vi "PhasedArrayRadar.vi"() -> ()   [LabVIEW 2015]
doc: "This example demonstrates how to use the Short-time Fourier Transform (STFT Spectrograms) VI to analyze the Time-Frequency spectrogram."
uses:
  <vilib>/Math Plots/3D Math Plots/3D Surface/3D Surface XCtrl/3D Surface.xctl
  <vilib>/sound2/lvsound2.llb/Sampling Mode.ctl
  <vilib>/Analysis/baseanly.llb/Mean (DBL).vi
  <vilib>/Analysis/2dsp.llb/Real FFT.vi
  <vilib>/Utility/file.llb/Read Delimited Spreadsheet (I64).vi
  <vilib>/Analysis/Matrix/Numeric/Conversions/Array To Matrix - RA.vi
  <vilib>/Analysis/Matrix/Numeric/Multiply/Multiply - RM,RM.vi
  <vilib>/Analysis/Matrix/Numeric/Conversions/Matrix To Array - RM.vi
  <vilib>/sound2/lvsound2.llb/Sound Input Read (DBL).vi
  <vilib>/Math Plots/3D Math Plots/3D Surface/3D Surface Datatype/Public/Plot Helper (Matrix).vi
  <vilib>/Analysis/NI_AALPro.lvlib
  <vilib>/Analysis/NI_AALBase.lvlib
  <vilib>/Math Plots/3D Math Plots/3D Surface/3D Surface Datatype/3D Surface Datatype.lvclass
  <vilib>/Analysis/Matrix/NI_Matrix.lvlib
panel:
  in  "Chirp repetition frequency":dbl=124.0
  in  "Save processed data":bool
  in  "Save raw data":bool
  in  "Data saving path":path=path "C:/Users/zpeng/OneDrive - Texas Tech University/Desktop/BeamSteering/data"
  out "3D Surface":refnum<class "3D Plot Datatype.lvclass">[](xcontrol)
  in  "Beam steering calibration data path":path=path "C:/Users/zpeng/OneDrive - Texas Tech University/Desktop/BeamSteering/voltages"
  in  "Angle step":dbl=2.5
  in  "Angle start":dbl=-60.0
  in  "Angle stop":dbl=60.0
  in  "Duty ratio":dbl=0.4
  in  "begin offsets":i32=548
  in  "end offsets":i32=562
  in  "Range":dbl(slide)=5.101767831965583 min=1.0 max=77.41935483870968 scale=0.0..77.41935483870968
  out "Range resolution":dbl
  in  "Bandwidth (MHz)":dbl=600.0
  in  "Range intensify:Minimum":dbl=-40.0
  out "Chirp frequency":dbl
  in  "FFT length":i32=4096
  out "Samples per chirp":i32
  in  "threshold":dbl=0.6 format="%0.2f"
  in  "Sample rate (S/s)":dbl=192000.0
  in  "Samples per read":i32=40000 min=1024 max=100000
  in  "Device ID":u32
  # "Phased Array"
  # "Version: 3\nZhengyu Peng\nC. Li Lab\nTexas Tech University\nJan. 2016"
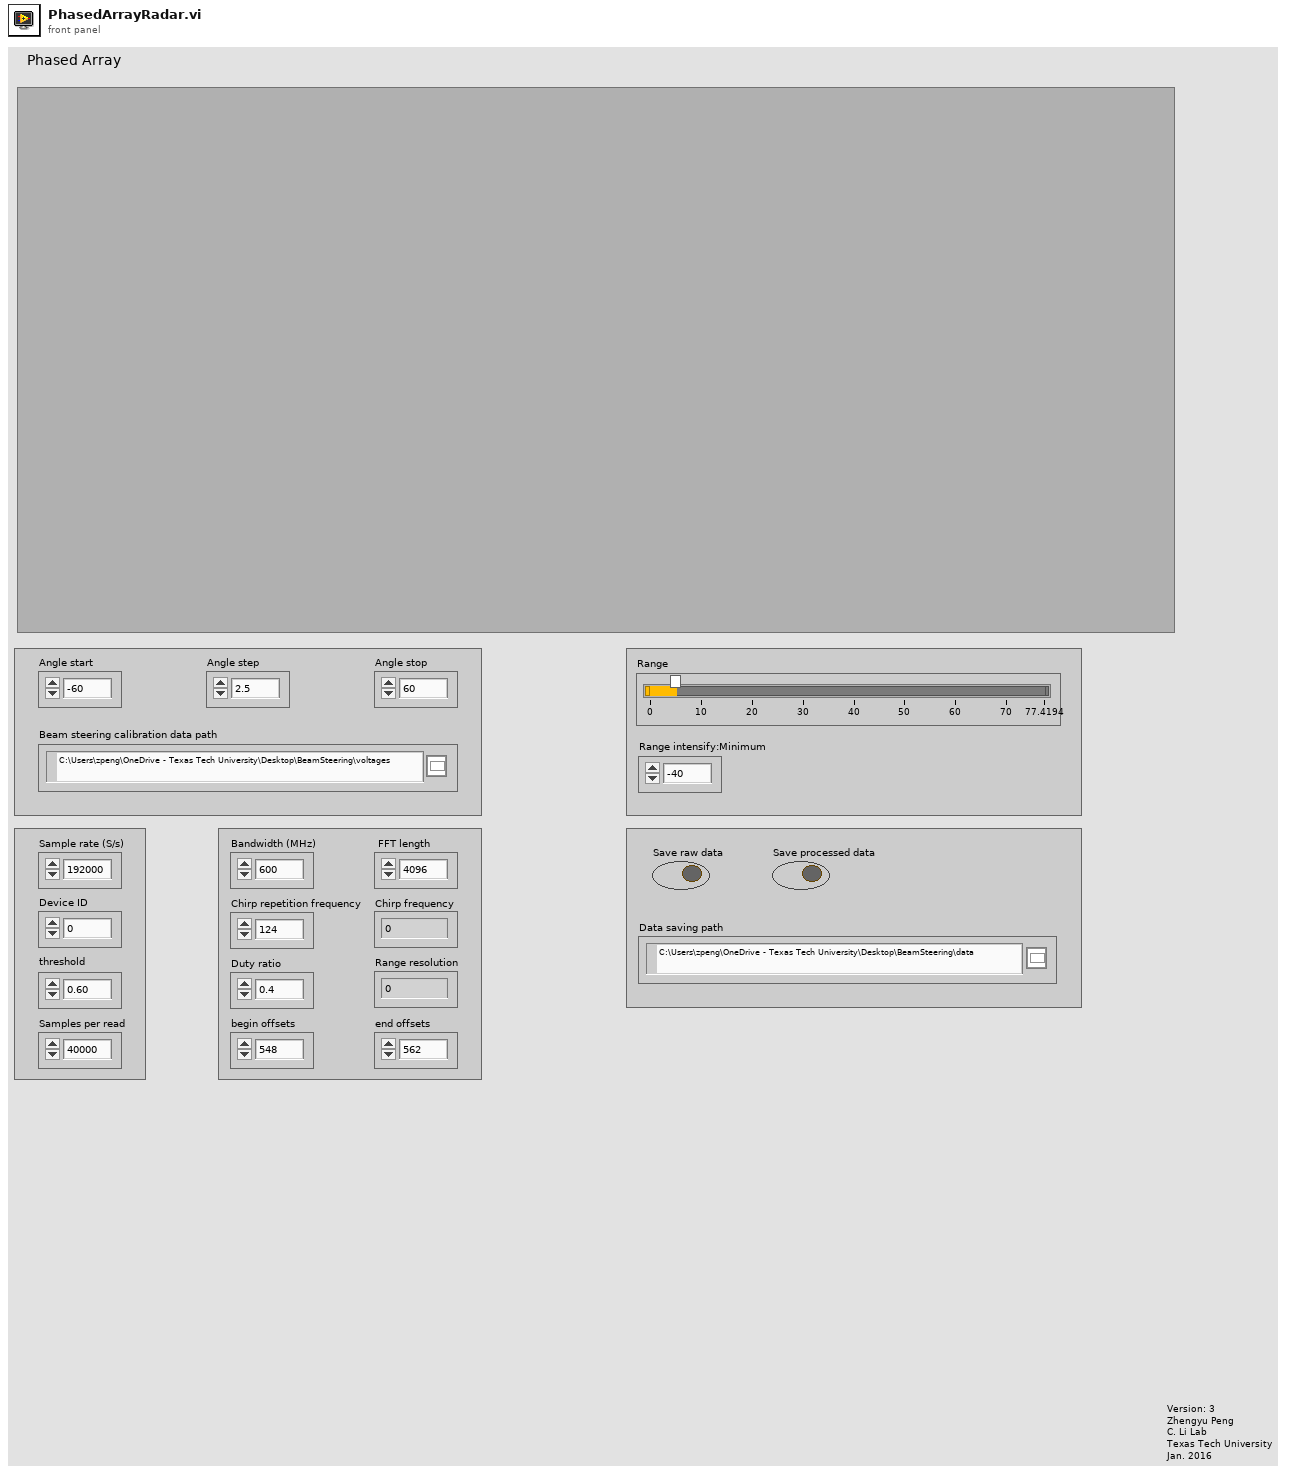
[diagram p1: front panel]
types:
  T1 = cluster{"Sample rate (S/s)":dbl, "number of channels":i32, "bits per sample":i32}
  T2 = typedef "NI_Matrix.lvlib/RealMatrix.ctl" = dbl[][]
  T3 = typedef "Sampling Mode.ctl" = i32
  T4 = typedef "Sound Input Task ID.ctl" = u32
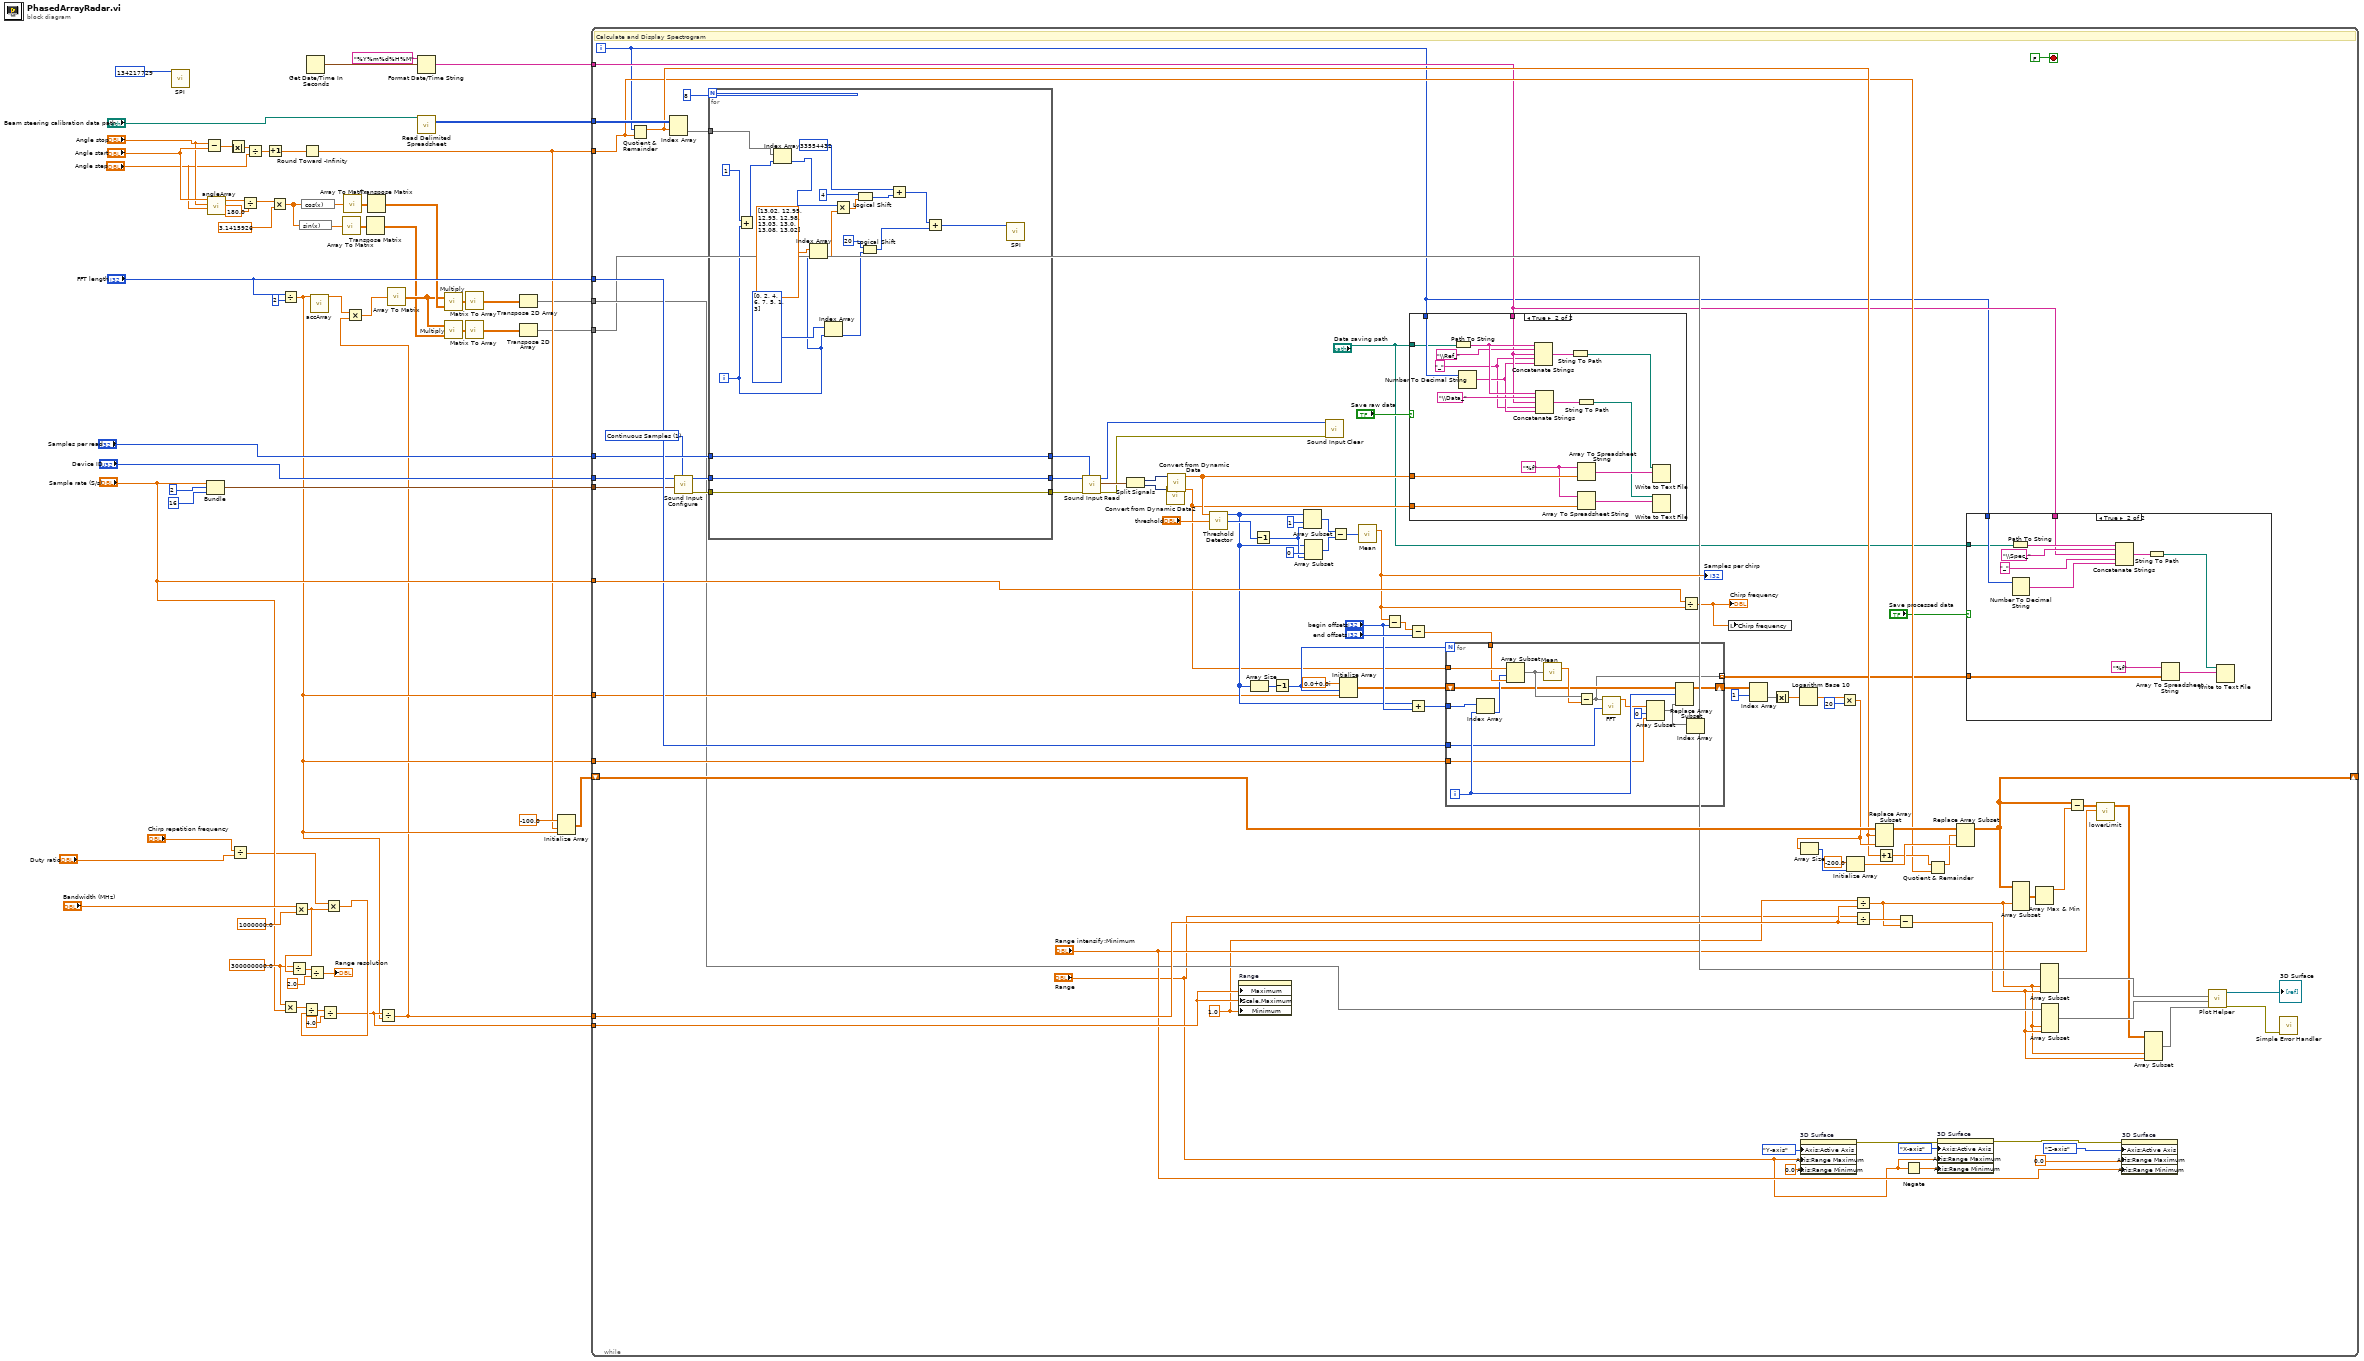
[diagram p0: block diagram]
diagram:
  w54 = 300000000.0 ("x")
  n1 = call "SPI.vi"("data"=u32 134217729) -> ()  [unwired: 11 in]
  n2 = Subtract(x="Angle stop", y="Angle start") -> (x-y=w41:dbl)
  n3 = Bundle("Sample rate (S/s)"="Sample rate (S/s)", "number of channels"=2, "bits per sample"=16) -> (w33:T1)  [unwired: 1 in]
  n4 = call "angleArray.vi"("Angle step"="Angle step", "Angle stop"="Angle stop", "Angle start"="Angle start") -> ("Array"=w26:dbl[])  [unwired: 8 in]
  n5 = Absolute Value(x=w41) -> (abs(x)=w40:dbl)
  n6 = Divide(x="Chirp repetition frequency", y="Duty ratio") -> (x/y=w45:dbl)
  n7 = Divide(x=w26, y=180.0) -> (x/y=w24:dbl[])
  n8 = Divide(x=w40, y="Angle step") -> (x/y=w39:dbl)
  n9 = Increment(x=w39) -> (x+1=w38:dbl)
  n10 = Multiply(x=w24, y=3.1415926) -> (x*y=w22:dbl[])
  n11 = Divide(x="FFT length", y=2) -> (x/y=w27:dbl)
  n12 = Multiply(x=w54, y="Sample rate (S/s)") -> (x*y=w53:dbl)
  n13 = Multiply(x="Bandwidth (MHz)", y=1000000.0) -> (x*y=w58:dbl)
  n14 = Divide(x=w54, y=w58) -> (x/y=w57:dbl)
  n15 = expression code="sin(x)"(w22) -> (w20:dbl[])
  n16 = expression code="cos(x)"(w22) -> (w21:dbl[])
  n17 = Round Toward -Infinity(1:w38) -> (0:w31:dbl)
  n18 = Get Date/Time In Seconds() -> (seconds since 1Jan1904=w4:timestamp)
  n19 = Divide(x=w57, y=2.0) -> (x/y=→"Range resolution":dbl)
  n20 = call "accArray.vi"("data length"=w27) -> ("Array"=w7:dbl[])  [unwired: 10 in]
  n21 = Multiply(x=w45, y=w58) -> (x*y=w52:dbl)
  n22 = Divide(x=w53, y=w52) -> (x/y=w51:dbl)
  n23 = Divide(x=w51, y=4.0) -> (x/y=w46:dbl)
  n24 = call-poly <vilib>:"Array To Matrix.vi"("Real 1D Array"=w20) -> ("Real Matrix (Column Vector)"=w18:T2)
  n25 = call-poly <vilib>:"Array To Matrix.vi"("Real 1D Array"=w21) -> ("Real Matrix (Column Vector)"=w19:T2)
  n26 = Transpose Matrix(1:w18) -> (0:w15:T2)
  n27 = Transpose Matrix(1:w19) -> (0:w17:T2)
  n28 = Divide(x=w46, y=w27) -> (x/y=w8:dbl)
  n29 = Multiply(x=w7, y=w8) -> (x*y=w6:dbl[])
  n30 = call-poly <vilib>:"Array To Matrix.vi"("Real 1D Array"=w6) -> ("Real Matrix (Column Vector)"=w16:T2)
  n31 = Format Date/Time String(time format string (%c)="%Y%m%d%H%M", seconds (now)=w4) -> (date/time string=w2:string)  [unwired: 1 in]
  n32 = call-poly <vilib>:"Read Delimited Spreadsheet.vi"("file path (dialog if empty)"="Beam steering calibration data path") -> ("all rows"=w35:i64[][])  [unwired: 9 in, 5 out]
  n33 = call-poly <vilib>:"Multiply.vi"("Real Matrix B"=w17, "Real Matrix A"=w16) -> ("A * B"=w14:T2)
  n34 = call-poly <vilib>:"Multiply.vi"("Real Matrix B"=w15, "Real Matrix A"=w16) -> ("A * B"=w13:T2)
  n35 = call-poly <vilib>:"Matrix To Array.vi"("Real Matrix"=w14) -> ("Real 2D Array"=w12:dbl[][])
  n36 = call-poly <vilib>:"Matrix To Array.vi"("Real Matrix"=w13) -> ("Real 2D Array"=w10:dbl[][])
  n37 = Transpose 2D Array(2D array=w12) -> (transposed array=w11:dbl[][])
  n38 = Transpose 2D Array(2D array=w10) -> (transposed array=w9:dbl[][])
  n39 = Initialize Array(-100.0 ("element"), w31, w27) -> (w32:dbl[][])
  n40 = while {
    tunnel: "Device ID" -> [w115]
    tunnel: "Samples per read" -> [w120]
    tunnel: "Sample rate (S/s)" -> [w142]
    tunnel: "FFT length" -> [w141]
    tunnel: w8 -> [w106]
    tunnel: w27 -> [w140]
    tunnel: w46 -> [w139]
    tunnel: w27 -> [w127]
    tunnel: w31 -> [w77]
    tunnel: w35 -> [w122]
    shift-right: [w79] -> _
    shift-left: w32 -> [w116]
    tunnel: w33 -> [w112]
    tunnel: w11 -> [w104]
    tunnel: w9 -> [w103]
    tunnel: w2 -> [w65]
    i -> [w64]
    stop <- FALSE stop-if-true
    w72 = T3 1 items=["Finite Samples", "Continuous Samples"] ("sample mode")
    w86 = 1.0 ("Data Entry Limits:Minimum")
    # "Calculate and Display Spectrogram"
    n41 = Quotient & Remainder(x=w64, y=w77) -> (x-y*floor(x/y)=w81:dbl)  [unwired: 1 out]
    n42 = Index Array(array=w122, index (row)=w81) -> (element=w123:i64[])  [unwired: 1 in]
    n43 = call <vilib>:"Sound Input Configure.vi"("sample mode"=w72, "sound format"=w112, "device ID"=w115) -> ("error out"=w113:errorcluster, "task ID"=w114:T4)  [unwired: 7 in]
    n44 = for {
      N: 8 -> [_]
      tunnel: w123 -> [w194]
      tunnel: [w187] -> w121
      tunnel: w114 -> [w187]
      tunnel: [w186] -> w119
      tunnel: w120 -> [w186]
      tunnel: [w185] -> w118
      tunnel: w113 -> [w185]
      i -> [w188]
      n45 = Add(x=1 ("length"), y=w188) -> (x+y=w193:i32)
      n46 = Index Array(array=w194, index=w193) -> (element=w192:i64)
      n47 = Index Array(array=dbl[] [13.02, 12.95, 12.93, 12.98, 13.03, 13.0, 13.08, 13.02] ("y"), index=w188) -> (element=w189:dbl)
      n48 = Index Array(array=i32[] [0, 2, 4, 6, 7, 5, 1, 3], index=w188) -> (element=w191:i32)
      n49 = Multiply(x=w192, y=w189) -> (x*y=w198:dbl)
      n50 = Logical Shift(y=u32 4 ("x"), x=w198) -> (x << y=w203:u32)
      n51 = Logical Shift(y=u32 20 ("x"), x=w191) -> (x << y=w201:i32)
      n52 = Add(x=u32 33554432 ("y"), y=w203) -> (x+y=w202:u32)
      n53 = Add(x=w202, y=w201) -> (x+y=w200:u32)
      n54 = call "SPI.vi"("data"=w200) -> ()  [unwired: 11 in]
    }
    n55 = call-poly <vilib>:"Sound Input Read.vi"("number of samples/ch"=w119, "error in (no error)"=w118, "task ID"=w121) -> ("error out"=w108:errorcluster, "data"=w153:waveform(dbl)[], "task ID out"=w111:T4)  [unwired: 6 in]
    n56 = Split Signals(w153) -> (w155:dynamicdata, w154:dynamicdata)  [unwired: 2 out]
    n57 = call "Convert from Dynamic Data2"("Dynamic Data Type"=w154) -> ("Array"=w69:dbl[])  [unwired: 3 out]
    n58 = call "Convert from Dynamic Data"("Dynamic Data Type"=w155) -> ("Array"=w70:dbl[])  [unwired: 3 out]
    n59 = call <vilib>:"Threshold Detector.vi"("threshold"="threshold", "X"=w70) -> ("count"=w148:i32, "Indices"=w131:i32[])  [unwired: 1 in, 1 out]
    n60 = property on="Range" class="Slide (strict)"("Maximum"=w139, "Scale.Maximum"=w139, "Minimum"=w86) -> ()  [unwired: 2 in, 2 out]
    n61 = Array Size(array=w131) -> (size(s)=w130:i32)
    n62 = Decrement(x=w148) -> (x-1=w147:i32)
    n63 = Decrement(x=w130) -> (x-1=w128:i32)
    n64 = Array Subset(array=w131, index=1, length=w147) -> (w150:i32[])
    n65 = Array Subset(array=w131, index=0, length=w147) -> (w149:i32[])
    n66 = call <vilib>:"Sound Input Clear.vi"("error in (no error)"=w108, "task ID"=w111) -> ()  [unwired: 9 in, 1 out]
    n67 = Subtract(x=w150, y=w149) -> (x-y=w146:i32[])
    n68 = Initialize Array(cdb 0.0+0.0i ("element"), w128, w127) -> (w126:cdb[][])
    n69 = call-poly <vilib>:"Mean.vi"("X"=w146) -> ("mean"=w135:dbl)  [unwired: 1 out]
    "Samples per chirp" <- w135
    n70 = Subtract(x=w135, y="begin offsets") -> (x-y=w133:dbl)
    n71 = case shown="True" "Save raw data" {
      tunnel: w70 -> [_ w184]
      tunnel: w64 -> [_ w182]
      tunnel: w69 -> [_ w177]
      tunnel: w65 -> [_ w171]
      tunnel: "Data saving path" -> [_ w168]
      frame False {
      }
      frame True {
        w169 = "_" ("string")
        w178 = "%f" ("format string")
        n72 = Path To String(path=w168) -> (string=w180:string)
        n73 = Number To Decimal String(number=w182) -> (decimal integer string=w170:string)  [unwired: 1 in]
        n74 = Concatenate Strings(w180, "\\Ref_" ("string"), w171, w169, w170) -> (w183:string)
        n75 = Concatenate Strings(w180, "\\Data_" ("string"), w171, w169, w170) -> (w179:string)
        n76 = String To Path(string=w183) -> (path=w175:path)
        n77 = Array To Spreadsheet String(array=w184, 3:w178) -> (spreadsheet string=w181:string)  [unwired: 1 in]
        n78 = Array To Spreadsheet String(array=w177, 3:w178) -> (spreadsheet string=w176:string)  [unwired: 1 in]
        n79 = String To Path(string=w179) -> (path=w174:path)
        n80 = Write to Text File(file (use dialog)=w175, text=w181) -> ()  [unwired: 2 in, 3 out]
        n81 = Write to Text File(file (use dialog)=w174, text=w176) -> ()  [unwired: 2 in, 3 out]
      }
    }
    n82 = Subtract(x=w133, y="end offsets") -> (x-y=w137:dbl)
    n83 = Add(x=w131, y="begin offsets") -> (x+y=w138:i32[])
    n84 = for {
      N: w128 -> [_]
      tunnel: w69 -> [w219]
      tunnel: w137 -> [w218]
      tunnel: w138 -> [w217]
      shift-right: [w215] -> w66
      shift-left: w126 -> [w206]
      tunnel: w141 -> [w213]
      tunnel: w140 -> [w208]
      tunnel: [w205] -> w62 mode=indexing
      i -> [w214]
      n85 = Index Array(array=w217, index=w214) -> (element=w216:i32)
      n86 = Array Subset(array=w219, index=w216, length=w218) -> (w212:dbl[])
      n87 = call-poly <vilib>:"Mean.vi"("X"=w212) -> ("mean"=w211:dbl)  [unwired: 1 out]
      n88 = Subtract(x=w212, y=w211) -> (x-y=w205:dbl[])
      n89 = call-poly <vilib>:"FFT.vi"("FFT size"=w213, "X"=w205) -> ("FFT {X}"=w210:cdb[])  [unwired: 8 in, 1 out]
      n90 = Array Subset(array=w210, index=0, length=w208) -> (w207:cdb[])
      n91 = Replace Array Subset(array=w206, new element=w207, index (row)=w214) -> (w215:cdb[][])  [unwired: 1 in]
      n92 = Index Array(array=w207) -> ()  [unwired: 1 in, 1 out]
    }
    n93 = Divide(x=w142, y=w135) -> (x/y=w71:dbl)
    "Chirp frequency" <- w71
    n94 = local write "Chirp frequency"(w71) -> ()
    n95 = Index Array(array=w66, index (row)=1) -> (element=w75:cdb[])  [unwired: 1 in]
    n96 = Absolute Value(x=w75) -> (abs(x)=w107:dbl[])
    n97 = Logarithm Base 10(1:w107) -> (0:w143:dbl[])
    n98 = property on="3D Surface" class="3D Surface (strict)"("Axis:Active Axis"=enum16{"X-axis", "Y-axis", "Z-axis"}."Y-axis", "Axis:Range Maximum"="Range", "Axis:Range Minimum"=sgl 0.0 ("Axis:Range:Range Minimum")) -> (error out=w96:errorcluster)  [unwired: 2 in, 1 out]
    n99 = Multiply(x=w143, y=i8 20 ("t")) -> (x*y=w84:dbl[])
    n100 = Array Size(array=w84) -> (size(s)=w83:i32)
    n101 = Initialize Array(-200.0 ("element"), w83) -> (w82:dbl[])
    n102 = Divide(x=w86, y=w106) -> (x/y=w100:dbl)
    n103 = Divide(x="Range", y=w106) -> (x/y=w105:dbl)
    n104 = Replace Array Subset(array=w116, new element=w84, index (row)=w81) -> (w80:dbl[][])  [unwired: 1 in]
    n105 = Increment(x=w81) -> (x+1=w78:dbl)
    n106 = Subtract(x=w105, y=w100) -> (x-y=w101:dbl)
    n107 = Negate(x="Range") -> (-x=w94:dbl)
    n108 = Quotient & Remainder(x=w78, y=w77) -> (x-y*floor(x/y)=w76:dbl)  [unwired: 1 out]
    n109 = property on="3D Surface" class="3D Surface (strict)"(error in=w96, "Axis:Active Axis"=enum16{"X-axis", "Y-axis", "Z-axis"}."X-axis", "Axis:Range Maximum"="Range", "Axis:Range Minimum"=w94) -> (error out=w92:errorcluster)  [unwired: 1 in, 1 out]
    n110 = Replace Array Subset(array=w80, new element=w82, index (row)=w76) -> (w79:dbl[][])  [unwired: 1 in]
    n111 = case shown="True" "Save processed data" {
      tunnel: w62 -> [_ w167]
      tunnel: w64 -> [_ w165]
      tunnel: w65 -> [_ w159]
      tunnel: "Data saving path" -> [_ w156]
      frame False {
      }
      frame True {
        n112 = Path To String(path=w156) -> (string=w163:string)
        n113 = Number To Decimal String(number=w165) -> (decimal integer string=w158:string)  [unwired: 1 in]
        n114 = Concatenate Strings(w163, "\\Spec_" ("string"), w159, "_" ("string"), w158) -> (w166:string)
        n115 = String To Path(string=w166) -> (path=w161:path)
        n116 = Array To Spreadsheet String(array=w167, 3:"%f" ("format string")) -> (spreadsheet string=w164:string)  [unwired: 1 in]
        n117 = Write to Text File(file (use dialog)=w161, text=w164) -> ()  [unwired: 2 in, 3 out]
      }
    }
    n118 = Array Subset(array=w79, index (col)=w100) -> (w132:dbl[][])  [unwired: 3 in]
    n119 = Array Max & Min(array=w132) -> (max value=w145:dbl)  [unwired: 3 out]
    n120 = Array Subset(array=w103, index (col)=w100, length (col)=w101) -> (w99:dbl[][])  [unwired: 2 in]
    n121 = Array Subset(array=w104, index (col)=w100, length (col)=w101) -> (w98:dbl[][])  [unwired: 2 in]
    n122 = Subtract(x=w79, y=w145) -> (x-y=w90:dbl[][])
    n123 = call "lowerLimit.vi"("Min"="Range intensify:Minimum", "data"=w90) -> ("output"=w89:dbl[][])  [unwired: 9 in]
    n124 = property on="3D Surface" class="3D Surface (strict)"(error in=w92, "Axis:Active Axis"=enum16{"X-axis", "Y-axis", "Z-axis"}."Z-axis", "Axis:Range Maximum"=sgl 0.0 ("Axis:Range:Range Maximum"), "Axis:Range Minimum"="Range intensify:Minimum") -> ()  [unwired: 1 in, 2 out]
    n125 = Array Subset(array=w89, index (col)=w100, length (col)=w101) -> (w102:dbl[][])  [unwired: 2 in]
    n126 = call-poly <vilib>:"Plot Helper.vi"("z matrix"=w102, "y matrix"=w98, "x matrix"=w99) -> ("error out"=w109:errorcluster, "3D Plot lvclass Array out"=→"3D Surface":refnum<class "3D Plot Datatype.lvclass">[])  [unwired: 4 in, 3 out]
    n127 = call <vilib>:"Simple Error Handler.vi"("error in (no error)"=w109) -> ()  [unwired: 4 in, 5 out]
  }
